vi "PKG_IMC_PropFollow.vi"(0 "handle":u32, 1 "srcEnd":i32, 2 "tgParam":i32, 3 "tgStart":i32, 5 "srcParam":i32, 7 "srcAxis":i32, 9 "srcStart":i32, 10 "id":i32, 12 "srcOffset":i32, 13 "tgAxis":i32, 14 "tgEnd":i32) -> (4 "handle out":u32, 6 "function return":i32)   [LabVIEW 2011, in "IMC_Pkg4xxx.lvlib"]
doc: "PKG_IMC_PropFollow(IMC_HANDLE handle, int srcParam, int srcAxis, int srcStart, int srcEnd, int srcOffset, int tgParam, int tgAxis, int tgStart, int tgEnd, int id);"
uses:
  IMC_Pkg4xxx.lvlib
  IMC_Pkg4xxx.dll
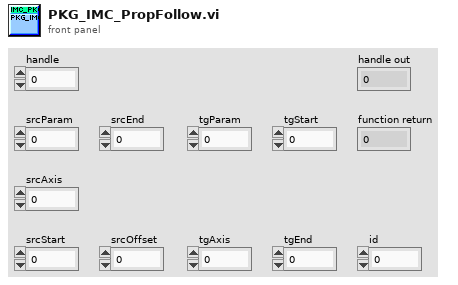
[diagram p1: front panel]
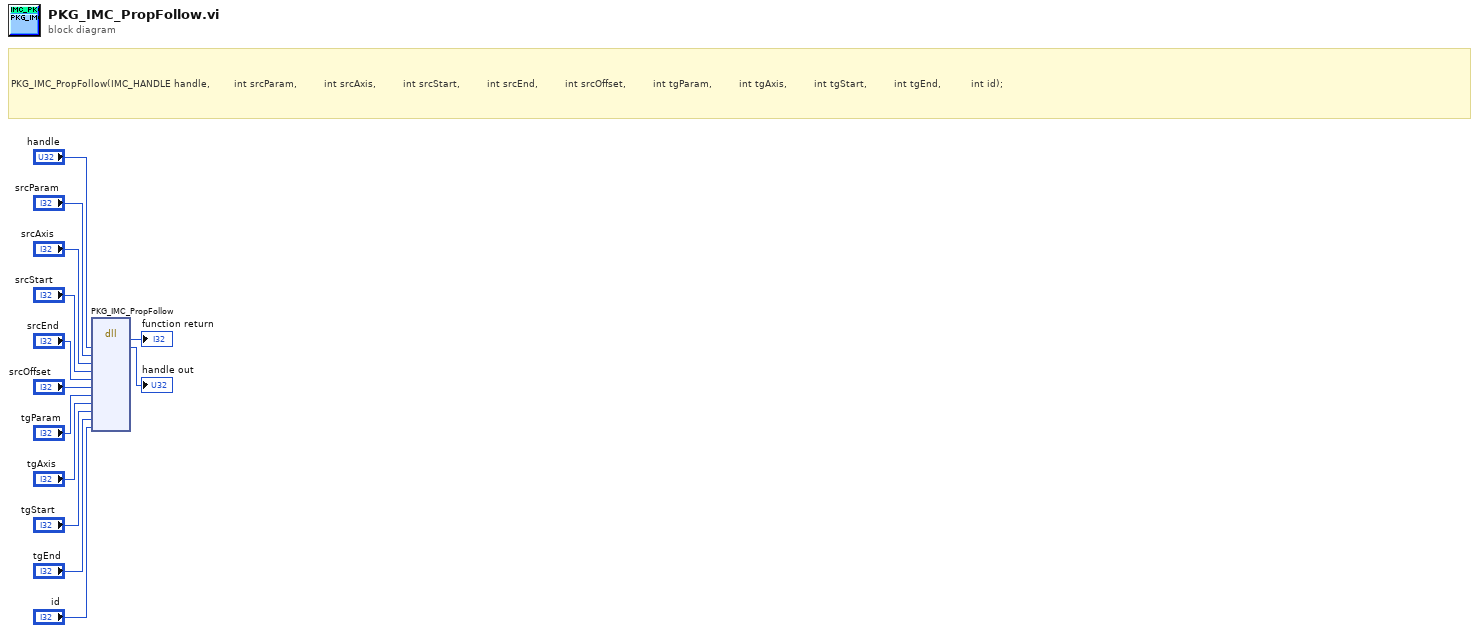
[diagram p0: block diagram]
diagram:
  # "PKG_IMC_PropFollow(IMC_HANDLE handle,  \t\t\t\t\t\tint srcParam, \t\t\t\t\t\t\t\tint srcAxis, \t\t\t\t\t\t\t\tint srcStart, \t\t\t\t\t\t\t\tint srcEnd, \t\t\t\t\t\t\t\tint srcOffset, \t\t\t\t\t\t\t\tint tgParam, \t\t\t\t\t\t\t\tint tgAxis, \t\t\t\t\t\t\t\tint tgStart, \t\t\t\t\t\t\t\tint tgEnd, \t\t\t\t\t\t\t\t\tint id);"
  n1 = dll-call lib="PTH1mabs F光盘刻录\niMC MotionIMCNet_V4.0IMCAppincLabviewIMC_PKG4xxxIMC_PKG4xxx\nIMC_Pkg4xxx.*" fn="PKG_IMC_PropFollow"("handle"="handle", "srcParam"="srcParam", "srcAxis"="srcAxis", "srcStart"="srcStart", "srcEnd"="srcEnd", "srcOffset"="srcOffset", "tgParam"="tgParam", "tgAxis"="tgAxis", "tgStart"="tgStart", "tgEnd"="tgEnd", "id"="id") -> (→"function return":i32, "handle"=→"handle out":u32)  [unwired: 13 in, 2 out]
